vi "Get Author Name.vi"(8 "error in (no error)":errorcluster, 11 "Demo Mouse in":refnum<class "Demo Mouse.lvclass">) -> (0 "error out":errorcluster, 2 "Author":string, 3 "Demo Mouse out":refnum<class "Demo Mouse.lvclass">)   [LabVIEW 2020, in "Demo.lvlib" / "Demo Mouse.lvclass"]
uses:
  Demo Mouse.lvclass
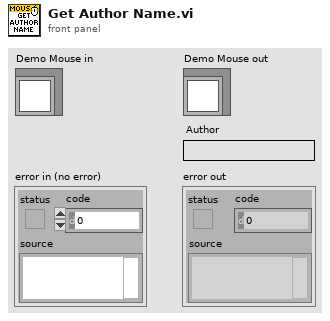
[diagram p1: front panel]
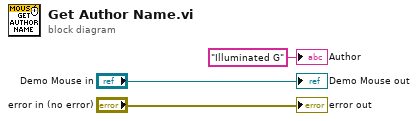
[diagram p0: block diagram]
diagram:
  "error out" <- "error in (no error)"
  "Demo Mouse out" <- "Demo Mouse in"
  "Author" <- "Illuminated G" ("Author")
